vi "st_Neg Binomial CDF (kx).vi"(9 "p":dbl=0.02, 10 "x":dbl=100.0, 11 "ky":dbl) -> (0 "error":i32, 3 "cdf(ky)":dbl=0.13261955589475294)   [LabVIEW 2024, in "NI_Gmath.lvlib"]
doc: "Computes the one-sided <B>probability</B>, p, of the normally distributed random variable, <B>x</B>."
uses:
  NI_Gmath.lvlib
  st_error_code.ctl
  Incomplete Beta Function.vi
panel:
  # "Negative Binomial CDF (ky)"
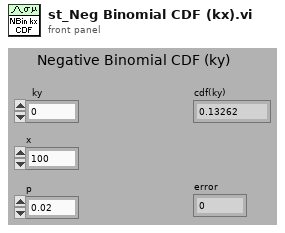
[diagram p1: front panel]
types:
  T1 = typedef "NI_Gmath.lvlib/st_error_code.ctl" = i32
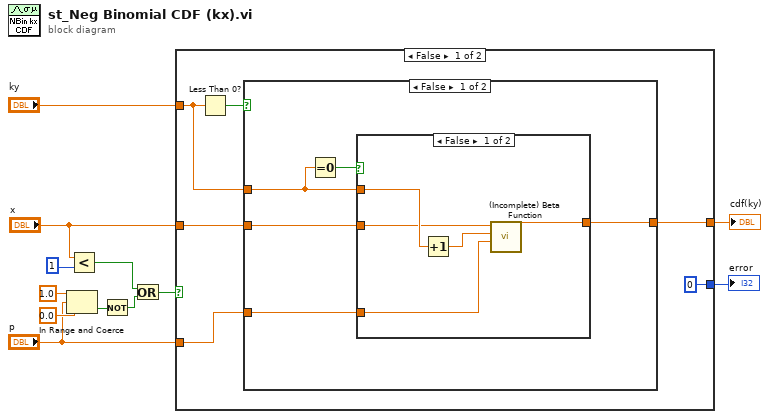
[diagram p0: block diagram]
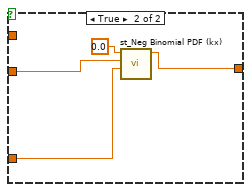
[diagram p2: hidden frame]
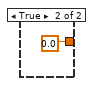
[diagram p3: hidden frame]
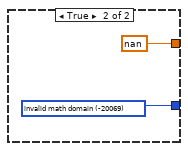
[diagram p4: hidden frame]
diagram:
  n1 = In Range and Coerce(upper limit=1.0, x="p", lower limit=0.0) -> (In Range?=w4:bool)  [unwired: 1 out]
  n2 = Less?(x="x", y=1) -> (x < y?=w2:bool)
  n3 = Not(x=w4) -> (.not. x?=w3:bool)
  n4 = Or(x=w2, y=w3) -> (x .or. y?=w7:bool)
  n5 = case shown="False" w7 {
    tunnel: [0 ("invalid math domain") w34] -> w12
    tunnel: [w17 nan] -> w11
    tunnel: "ky" -> [w13 _]
    tunnel: "x" -> [w16 _]
    tunnel: "p" -> [w15 _]
    frame False {
      n6 = Less Than 0?(x=w13) -> (x < 0?=w14:bool)
      n7 = case shown="False" w14 {
        tunnel: [w23 0.0] -> w17
        tunnel: w13 -> [w22 _]
        tunnel: w16 -> [w21 _]
        tunnel: w15 -> [w20 _]
        frame False {
          n8 = Equal To 0?(x=w22) -> (x = 0?=w19:bool)
          n9 = case shown="False" w19 {
            tunnel: w21 -> [w26 w30]
            tunnel: w20 -> [w24 w31]
            tunnel: [w25 w29] -> w23
            tunnel: w22 -> [w28 _]
            frame False {
              n10 = Increment(x=w28) -> (x+1=w27:dbl)
              n11 = call-poly "(Incomplete) Beta Function.vi"("a"=w24, "y"=w27, "x"=w26) -> ("b(x, y, a)"=w25:dbl)  [unwired: 8 in]
            }
            frame True {
              n12 = call "st_Neg Binomial PDF (kx).vi"("p"=w31, "x"=w30, "ky"=0.0 ("a")) -> ("pdf(ky)"=w29:dbl)  [unwired: 7 in, 1 out]
            }
          }
        }
        frame True {
        }
      }
    }
    frame True {
      w34 = T1 -20069 items=["invalid math domain"=-20069, "Fourier interpolation size m >= n"=-20070, "empty array"=-20003] ("stat interp error code")
    }
  }
  "cdf(ky)" <- w11
  "error" <- w12
